vi "ArrayNumeric.vi"() -> ()   [LabVIEW 2019]
panel:
  out "x+y":dbl[](array[numeric])
  in  "b":dbl[](array[numeric])
  in  "a":dbl[](array[numeric])
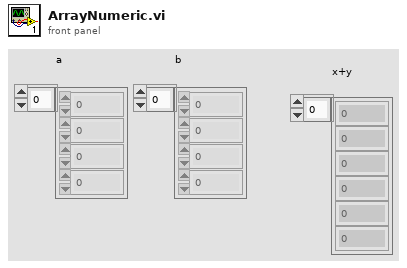
[diagram p1: front panel]
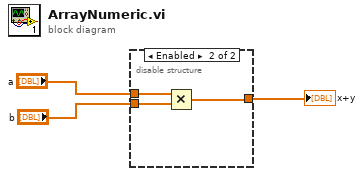
[diagram p0: block diagram]
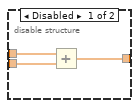
[diagram p2: hidden frame]
diagram:
  n1 = disable-structure shown="Enabled" {
    disable-tunnel: "a" -> [w6 w9]
    disable-tunnel: "b" -> [w5 w8]
    disable-tunnel: [w4 w7] -> w1
    frame Disabled {
      n2 = Add(x=w6, y=w5) -> (x+y=w4:dbl[])
    }
    frame Enabled {
      n3 = Multiply(x=w9, y=w8) -> (x*y=w7:dbl[])
    }
  }
  "x+y" <- w1
